vi "Set and Get Num of Rows Or Cols.vi"(6 "Row Or Col":T1=enum."Col", 7 "Mode":T2, 8 "错误输入":errorcluster, 10 "Number of Rows or Cols In":u32, 11 "Mlistbox Ref":refnum<vi>) -> (0 "错误输出":errorcluster, 2 "Number of Rows or Cols Out":u32, 3 "Mlistbox Ref Dup":refnum<vi>)   [LabVIEW 2012, in "Mlistbox Tools.lvlib"]
uses:
  Mlistbox Tools.lvlib
  ListBox/Custom Type/Read and Write Mode.ctl
  Custom Type/Row and Col Option.ctl
  ListBox/Listbox Tool.lvlib
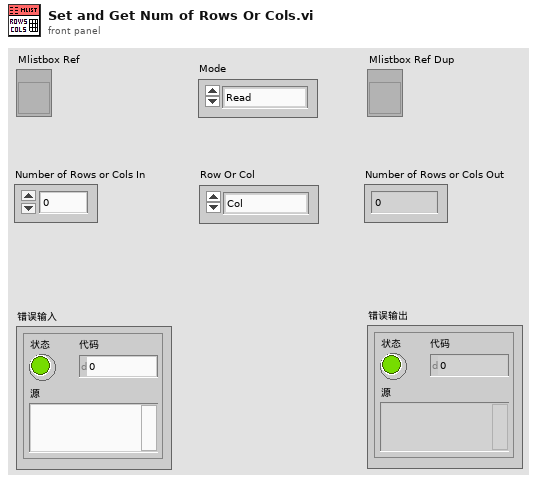
[diagram p1: front panel]
types:
  T1 = typedef "Mlistbox Tools.lvlib/Row and Col Option.ctl" = enum16{"Row", "Col"}
  T2 = typedef "Listbox Tool.lvlib/Read and Write Mode.ctl" = enum16{"Read", "Write"}
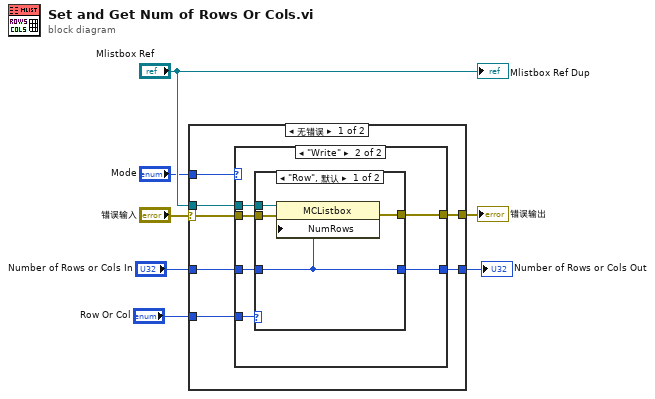
[diagram p0: block diagram]
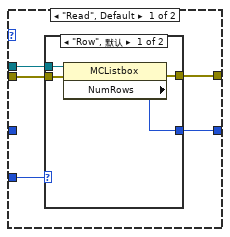
[diagram p2: hidden frame]
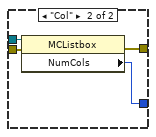
[diagram p3: hidden frame]
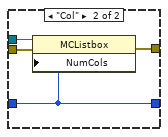
[diagram p4: hidden frame]
diagram:
  n1 = case shown="无错误" "错误输入" {
    selector: "错误输入" -> [w12 w42]
    tunnel: [w10 w42] -> w6
    tunnel: "Mlistbox Ref" -> [w13 _]
    tunnel: "Mode" -> [w14 _]
    tunnel: [w11 _] -> w2
    tunnel: "Number of Rows or Cols In" -> [w9 _]
    tunnel: "Row Or Col" -> [w8 _]
    frame No Error {
      n2 = case shown="\"Write\"" w14 {
        tunnel: w13 -> [w19 w33]
        tunnel: w12 -> [w18 w32]
        tunnel: [w17 w28] -> w11
        tunnel: [w16 w31] -> w10
        tunnel: w9 -> [_ w30]
        tunnel: w8 -> [w15 w29]
        frame "Read", Default {
          n3 = case shown="\"Row\", 默认" w15 {
            tunnel: w19 -> [w23 w27]
            tunnel: w18 -> [w22 w26]
            tunnel: [w20 w25] -> w17
            tunnel: [w21 w24] -> w16
            frame "Row", Default {
              n4 = property class="MCListbox"(reference=w23, error in=w22) -> (error out=w21:errorcluster, "NumRows"=w20:u32)  [unwired: 1 out]
            }
            frame "Col" {
              n5 = property class="MCListbox"(reference=w27, error in=w26) -> (error out=w24:errorcluster, "NumCols"=w25:u32)  [unwired: 1 out]
            }
          }
        }
        frame "Write" {
          n6 = case shown="\"Row\", 默认" w29 {
            tunnel: w33 -> [w36 w41]
            tunnel: w32 -> [w37 w40]
            tunnel: [w34 w39] -> w31
            tunnel: w30 -> [w35 w38]
            tunnel: [w35 w38] -> w28
            frame "Row", Default {
              n7 = property class="MCListbox"(reference=w36, error in=w37, "NumRows"=w35) -> (error out=w34:errorcluster)  [unwired: 1 out]
            }
            frame "Col" {
              n8 = property class="MCListbox"(reference=w41, error in=w40, "NumCols"=w38) -> (error out=w39:errorcluster)  [unwired: 1 out]
            }
          }
        }
      }
    }
    frame Error {
    }
  }
  "错误输出" <- w6
  "Number of Rows or Cols Out" <- w2
  "Mlistbox Ref Dup" <- "Mlistbox Ref"
